vi "外观.vi"(0 "Data In":T1 caption="数据输入", 2 "Display State In":T5={"功能选择"=enum."扫描", "扫描参数"={"+ V"=0.0, "+ Δ V"=0.0, "+ limit I"=0.01, "- V"=0.0, "- Δ V"=0.0, "- limit I"=0.01, "NPLC"=0.001, "模型"=FALSE}, "保持时间"={"V"=0.0, "limit I"=0.01, "T"=0.0, "ΔT"=0.0, "NPLC"=0.001}, "脉冲1"={"t0"=timestamp(0 s since 1904-01-01), "dt"=1.0, "Y"=[]}, "脉冲2"={"t0"=timestamp(0 s since 1904-01-01), "dt"=1.0, "Y"=[]}, "高速脉冲1"={"t0"=timestamp(0 s since 1904-01-01), "dt"=1.0, "Y"=[]}, "高速脉冲2"={"t0"=timestamp(0 s since 1904-01-01), "dt"=1.0, "Y"=[]}, "任意波形"={"t0"=timestamp(0 s since 1904-01-01), "dt"=1.0, "Y"=[]}} caption="显示状态输入" {"保持时间"."ΔT" min=0.5 max=100.0 step=0.1 format="%#_6ps"; "保持时间"."T" min=10.0 max=4294000.0 step=1.0 format="%#_6ps"; "保持时间"."NPLC" min=1.0 max=20.0 step=1.0; "保持时间"."limit I" min=1e-08 max=3.0 format="%#_6pA"; "保持时间"."V" min=-40.0 max=40.0 format="%#_6pV"; "扫描参数"."NPLC" min=0.001 max=25.0 step=0.001; "扫描参数"."- Δ V" min=5e-05 max=1.0 step=5e-05 format="%#_6pV"; "扫描参数"."+ Δ V" min=5e-05 max=1.0 step=5e-05 format="%#_6pV"; "扫描参数"."- V" min=-40.0 max=40.0 format="%#_6pV"; "扫描参数"."- limit I" min=1e-08 max=3.0 format="%#_6pA"; "扫描参数"."+ limit I" min=1e-08 max=3.0 format="%#_6pA"; "扫描参数"."+ V" min=-40.0 max=40.0 format="%#_6pV"}, 3 "Container State":T6 caption="容器状态") -> (6 "Data Out":T1 caption="数据输出", 7 "Display State Out":T5={"功能选择"=enum."扫描", "扫描参数"={"+ V"=0.0, "+ Δ V"=0.0, "+ limit I"=0.01, "- V"=0.0, "- Δ V"=0.0, "- limit I"=0.01, "NPLC"=0.001, "模型"=FALSE}, "保持时间"={"V"=0.0, "limit I"=0.01, "T"=0.0, "ΔT"=0.0, "NPLC"=0.001}, "脉冲1"={"t0"=timestamp(0 s since 1904-01-01), "dt"=1.0, "Y"=[]}, "脉冲2"={"t0"=timestamp(0 s since 1904-01-01), "dt"=1.0, "Y"=[]}, "高速脉冲1"={"t0"=timestamp(0 s since 1904-01-01), "dt"=1.0, "Y"=[]}, "高速脉冲2"={"t0"=timestamp(0 s since 1904-01-01), "dt"=1.0, "Y"=[]}, "任意波形"={"t0"=timestamp(0 s since 1904-01-01), "dt"=1.0, "Y"=[]}} caption="显示状态输出" {"保持时间"."ΔT" min=0.5 max=100.0 step=0.1 format="%#_6ps"; "保持时间"."T" min=10.0 max=4294000.0 step=1.0 format="%#_6ps"; "保持时间"."NPLC" min=1.0 max=20.0 step=1.0; "保持时间"."limit I" min=1e-08 max=3.0 format="%#_6pA"; "保持时间"."V" min=-40.0 max=40.0 format="%#_6pV"; "扫描参数"."NPLC" min=0.001 max=25.0 step=0.001; "扫描参数"."- Δ V" min=5e-05 max=1.0 step=5e-05 format="%#_6pV"; "扫描参数"."+ Δ V" min=5e-05 max=1.0 step=5e-05 format="%#_6pV"; "扫描参数"."- V" min=-40.0 max=40.0 format="%#_6pV"; "扫描参数"."- limit I" min=1e-08 max=3.0 format="%#_6pA"; "扫描参数"."+ limit I" min=1e-08 max=3.0 format="%#_6pA"; "扫描参数"."+ V" min=-40.0 max=40.0 format="%#_6pV"}, 8 "Action":T4 caption="动作")   [LabVIEW 2020, in "功能选择.xctl"]
uses:
  <vilib>/_xctls/Container State.ctl
  <vilib>/_xctls/Action.ctl
  <vilib>/_xctls/XControlSupport.lvlib
panel:
  in  "功能选择":T1
  out "选项卡控件":enum32{"扫描", "保持时间", "脉冲", "高速脉冲", "任意波形"}(tab)
  in  "扫描参数":T2={"+ V"=1.0, "+ Δ V"=0.01, "+ limit I"=0.01, "- V"=1.0, "- Δ V"=0.01, "- limit I"=0.01, "NPLC"=1.0, "模型"=FALSE} {"NPLC" min=0.001 max=25.0 step=0.001; "- Δ V" min=5e-05 max=1.0 step=5e-05 format="%#_6pV"; "+ Δ V" min=5e-05 max=1.0 step=5e-05 format="%#_6pV"; "- V" min=-40.0 max=40.0 format="%#_6pV"; "- limit I" min=1e-08 max=3.0 format="%#_6pA"; "+ limit I" min=1e-08 max=3.0 format="%#_6pA"; "+ V" min=-40.0 max=40.0 format="%#_6pV"}
  in  "保持时间":T3={"V"=0.1, "limit I"=0.01, "T"=10000.0, "ΔT"=1.0, "NPLC"=1.0} {"ΔT" min=0.5 max=100.0 step=0.1 format="%#_6ps"; "T" min=10.0 max=4294000.0 step=1.0 format="%#_6ps"; "NPLC" min=1.0 max=20.0 step=1.0; "limit I" min=1e-08 max=3.0 format="%#_6pA"; "V" min=-40.0 max=40.0 format="%#_6pV"}
  out "脉冲2":waveform(dbl)(graph)
  out "脉冲1":waveform(dbl)(graph)
  out "高速脉冲2":waveform(dbl)(graph) caption="脉冲2"
  out "高速脉冲1":waveform(dbl)(graph) caption="脉冲1"
  out "任意波形":waveform(dbl)(graph)
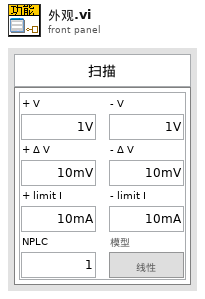
[diagram p1: front panel]
types:
  T1 = typedef "功能选择.xctl/功能类型选择.ctl" = enum16{"扫描", "循环扫描", "保持时间", "脉冲", "高速脉冲", "任意波形"}
  T2 = typedef "功能选择.xctl/扫描参数.ctl" = cluster{"+ V":dbl, "+ Δ V":dbl, "+ limit I":dbl, "- V":dbl, "- Δ V":dbl, "- limit I":dbl, "NPLC":dbl, "模型":bool}
  T3 = typedef "功能选择.xctl/保持时间.ctl" = cluster{"V":dbl, "limit I":dbl, "T":dbl, "ΔT":dbl, "NPLC":dbl}
  T4 = typedef "XControlSupport.lvlib/Action.ctl" = cluster{"Data Changed?":bool, "State Changed?":bool, "Action Name":string}
  T5 = typedef "功能选择.xctl/状态.ctl" = cluster{"功能选择":T1, "扫描参数":T2, "保持时间":T3, "脉冲1":waveform(dbl), "脉冲2":waveform(dbl), "高速脉冲1":waveform(dbl), "高速脉冲2":waveform(dbl), "任意波形":waveform(dbl)}
  T6 = typedef "XControlSupport.lvlib/Container State.ctl" = cluster{"Indicator?":bool, "Run Mode?":bool, " Refnum":refnum<vi>}
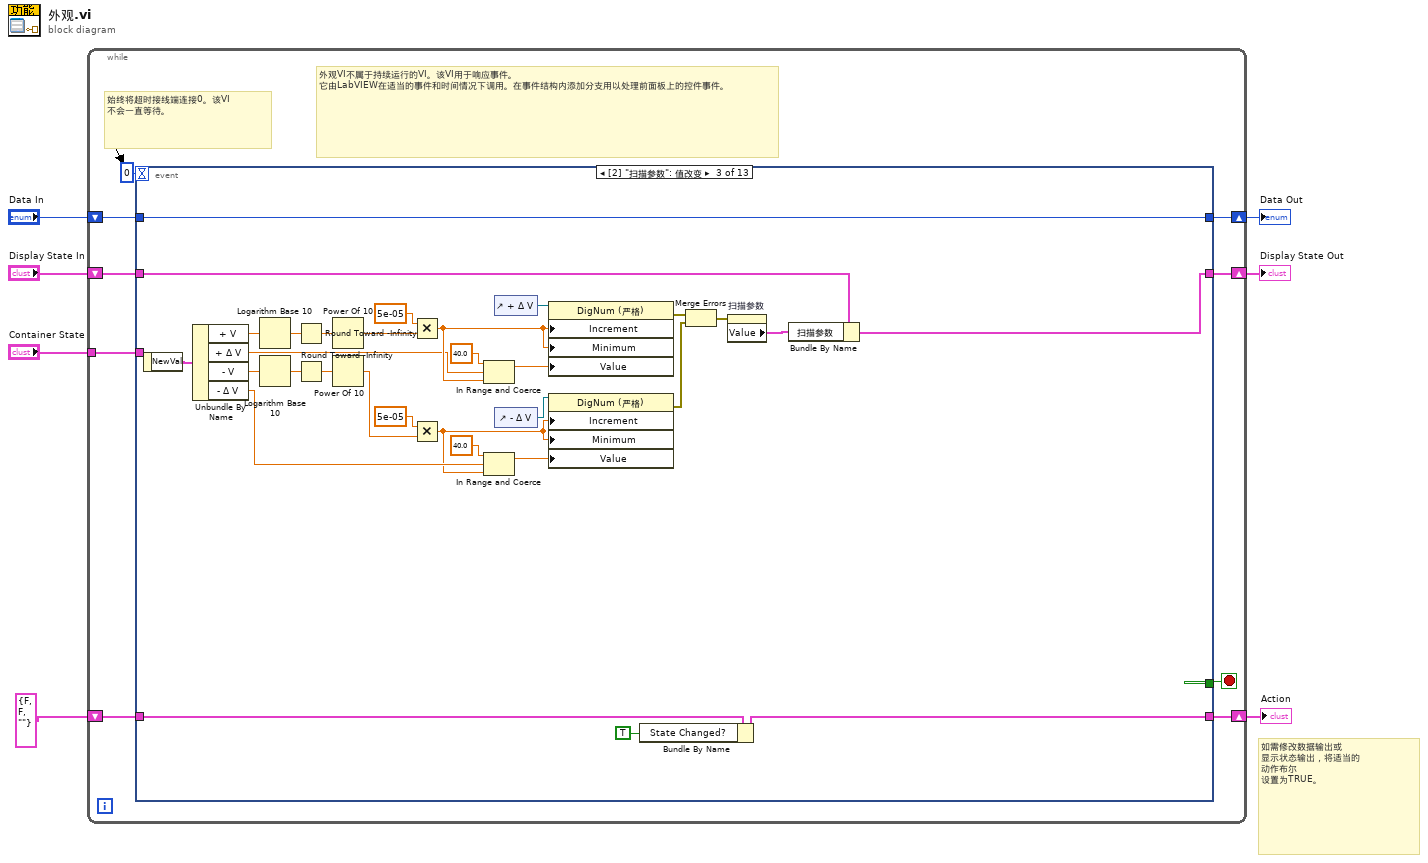
[diagram p0: block diagram]
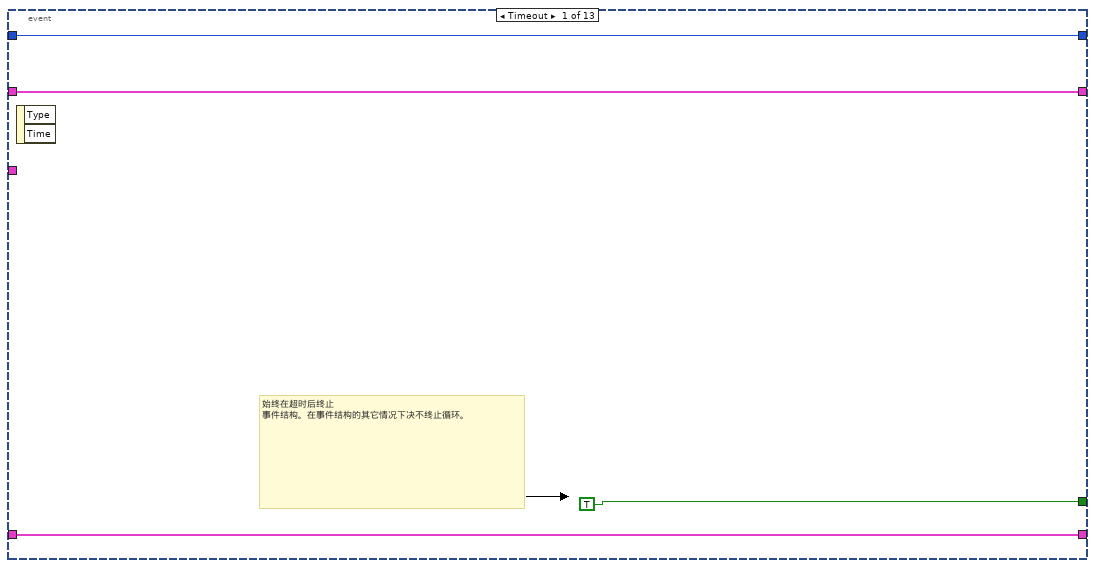
[diagram p2: hidden frame]
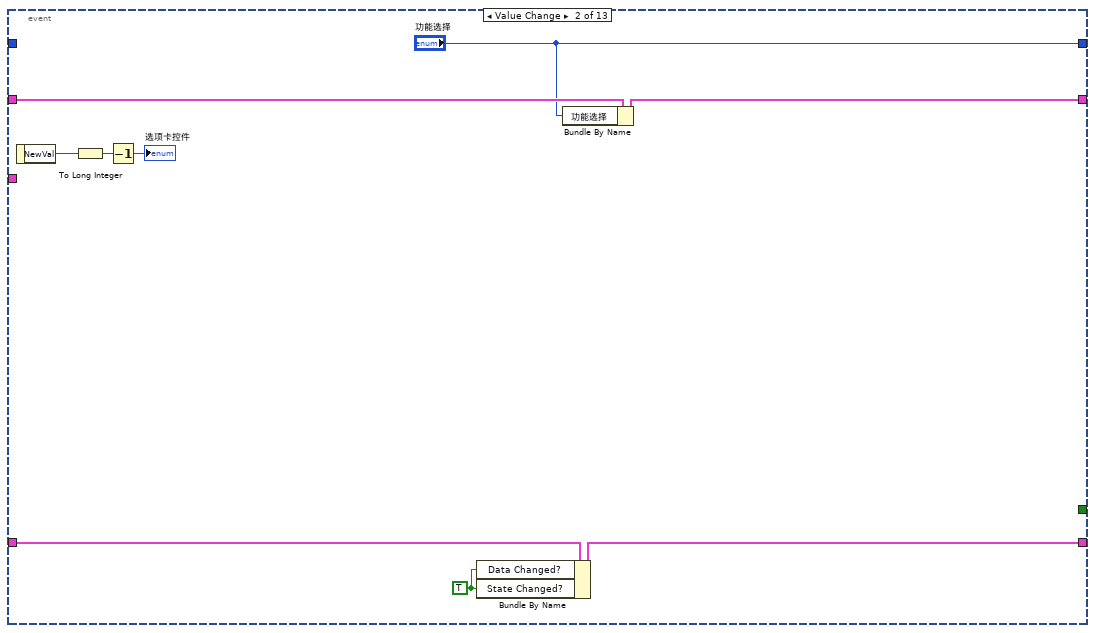
[diagram p3: hidden frame]
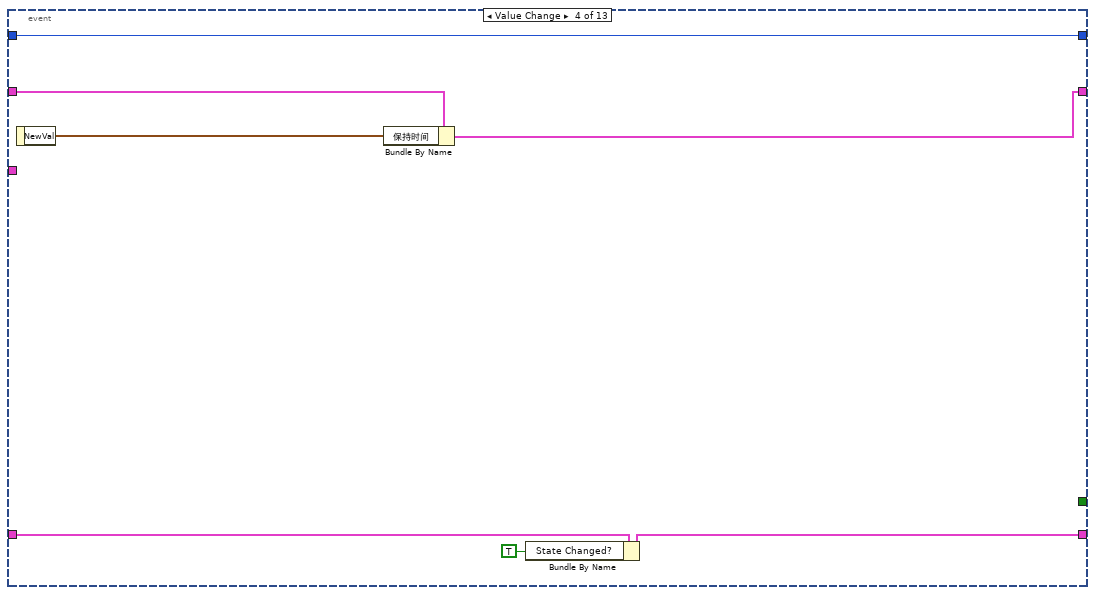
[diagram p4: hidden frame]
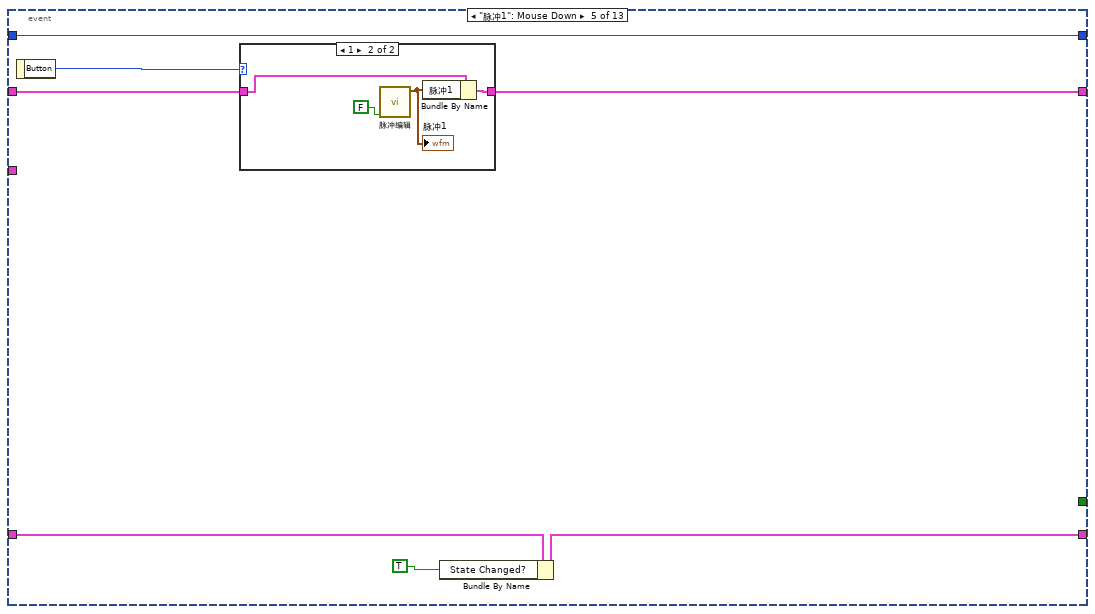
[diagram p5: hidden frame]
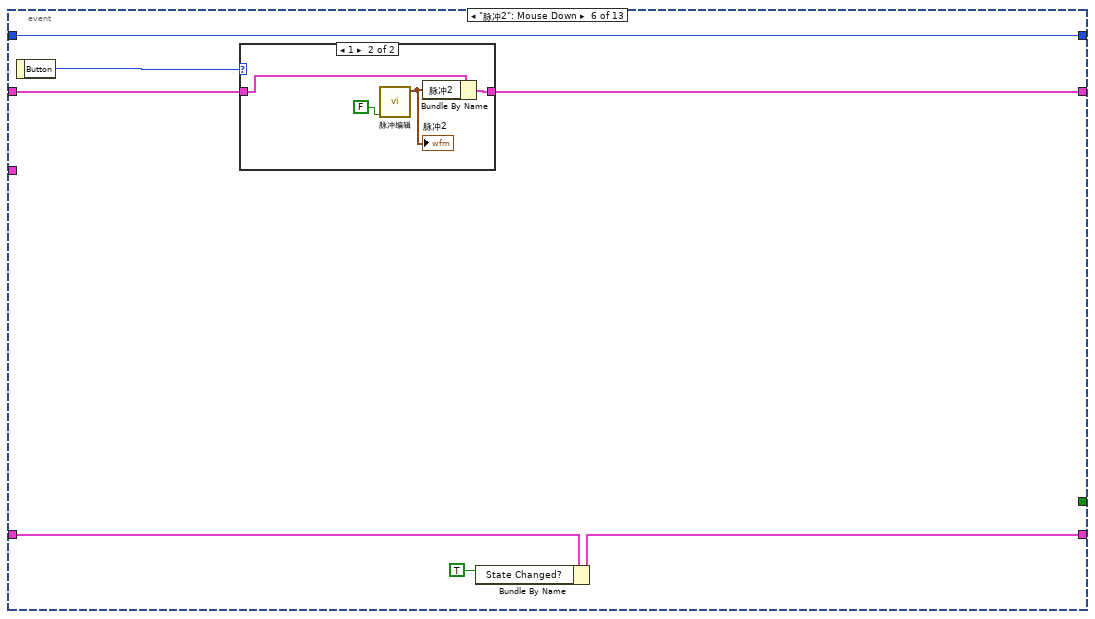
[diagram p7: hidden frame]
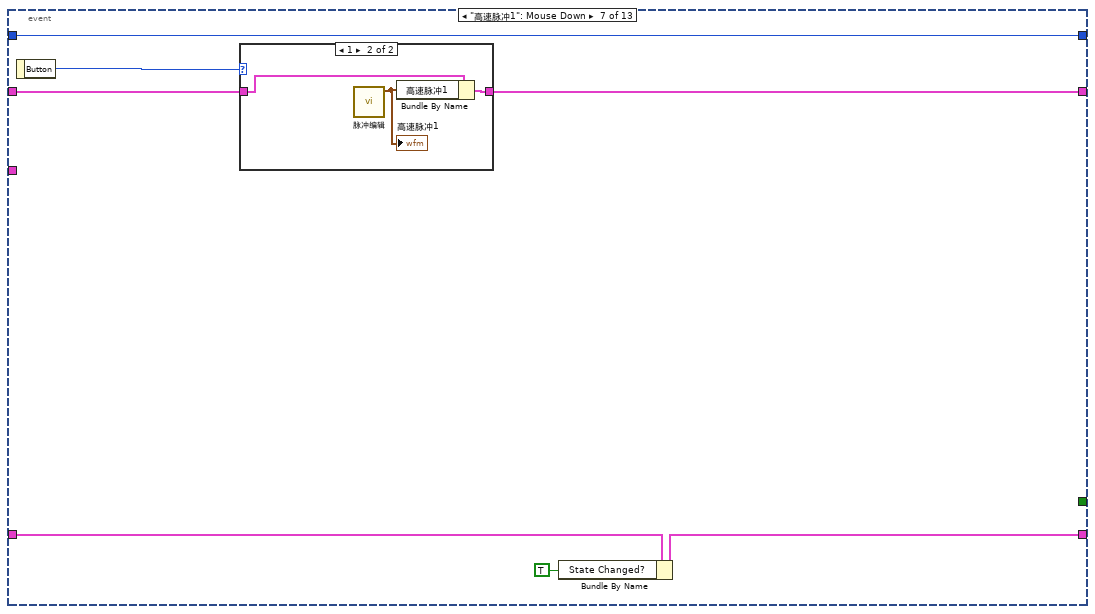
[diagram p9: hidden frame]
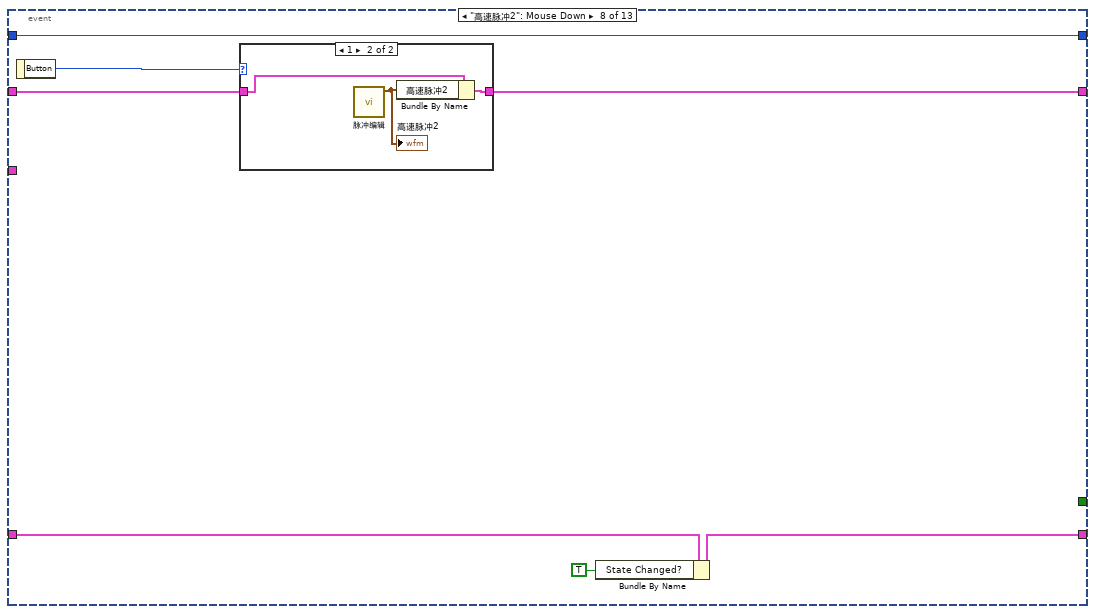
[diagram p11: hidden frame]
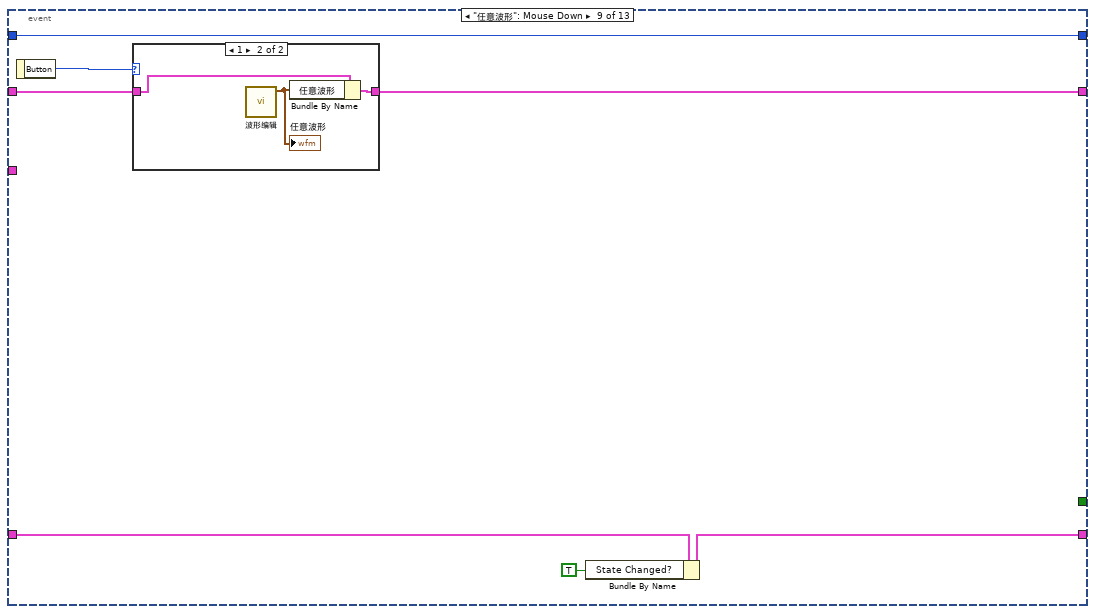
[diagram p13: hidden frame]
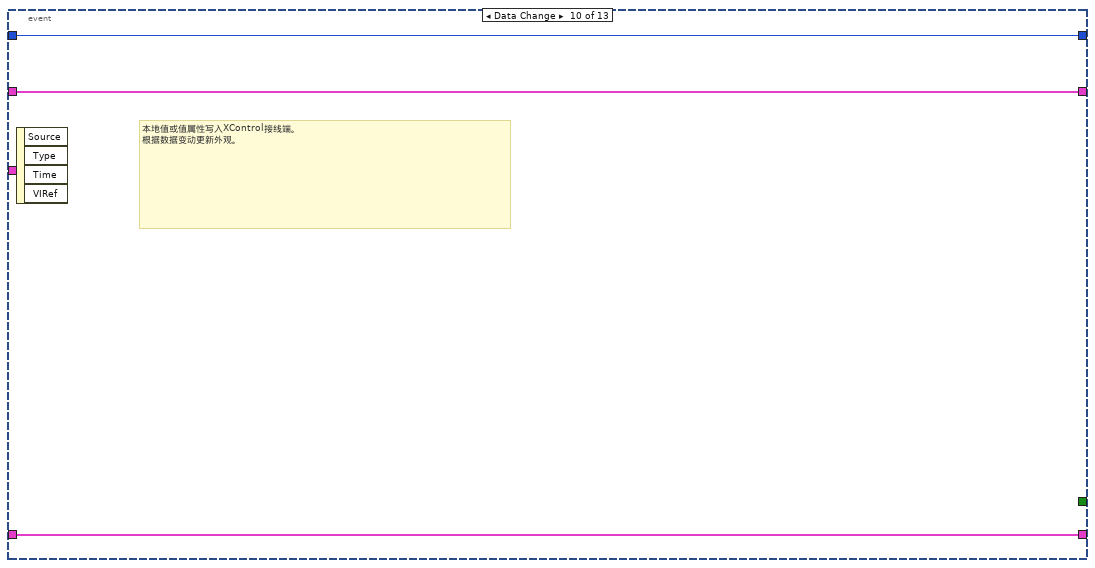
[diagram p15: hidden frame]
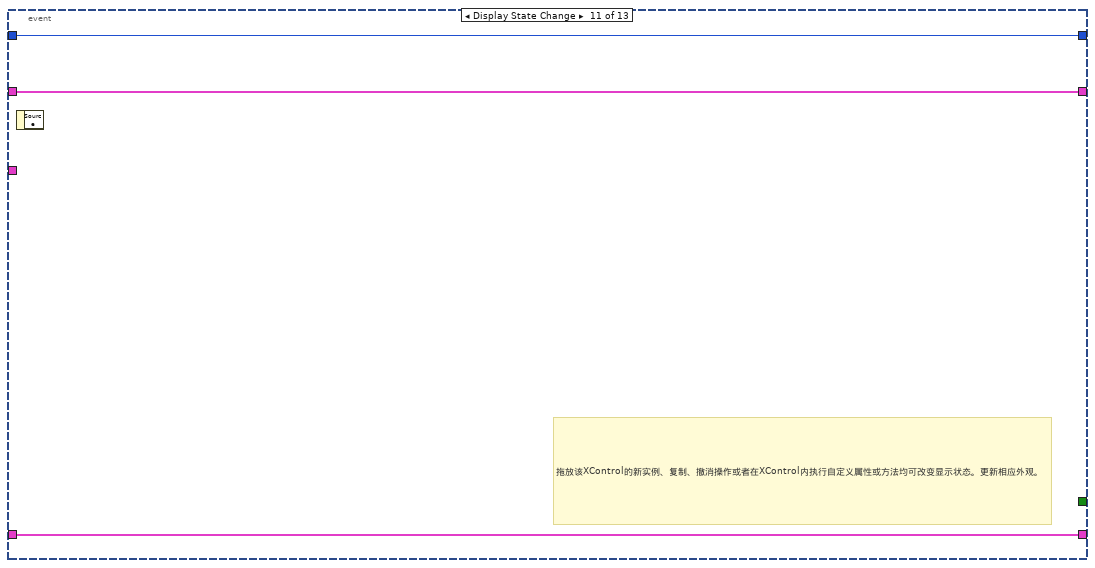
[diagram p16: hidden frame]
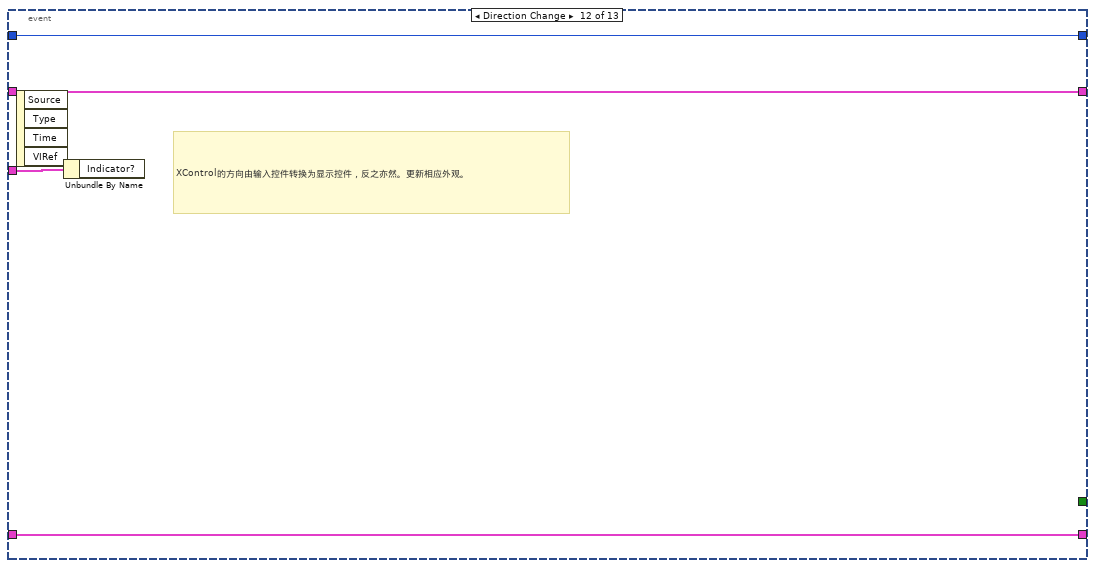
[diagram p17: hidden frame]
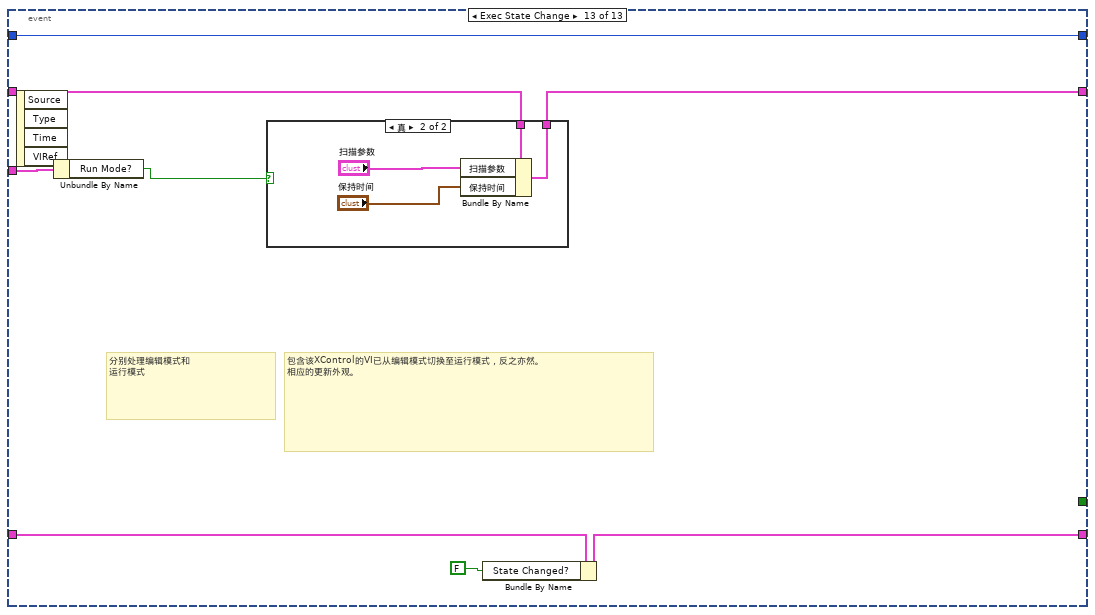
[diagram p18: hidden frame]
diagram:
  # "如需修改数据输出或\n显示状态输出，将适当的\n动作布尔\n设置为TRUE。"
  n1 = while {
    shift-right: [w15] -> w4
    shift-left: "Display State In" -> [w16]
    tunnel: "Container State" -> [w12]
    shift-right: [w10] -> w7
    shift-left: "Data In" -> [w11]
    shift-right: [w8] -> w2
    shift-left: T4 {"Data Changed?"=FALSE, "State Changed?"=FALSE, "Action Name"=""} ("Action") -> [w9]
    stop <- w14 stop-if-true
    # "外观VI不属于持续运行的VI。该VI用于响应事件。  它由LabVIEW在适当的事件和时间情况下调用。在事件结构内添加分支用以处理前面板上的控件事件。"
    # "始终将超时接线端连接0。该VI\n不会一直等待。"
    n2 = event shown="[2] \"扫描参数\": 值改变" {
      selector: _ -> [_ _ _ _ _ _ _ _ _ _ _ _ _]
      dyn-events: _ -> [_ _ _ _ _ _ _ _ _ _ _ _ _]
      timeout: 0 -> [_ _ _ _ _ _ _ _ _ _ _ _ _]
      tunnel: w16 -> [w18 w29 w60 w67 w72 w84 w96 w108 w116 w127 w129 w133 w141]
      tunnel: [w18 w25 w47 w63 w70 w82 w94 w106 w117 w127 w129 w133 w138] -> w15
      tunnel: [TRUE _ _ _ _ _ _ _ _ _ _ _ _] -> w14
      tunnel: w12 -> [_ _ _ _ _ _ _ _ _ _ _ w134 w142]
      tunnel: w11 -> [w17 _ w46 w66 w71 w83 w95 w107 w120 w126 w128 w132 w140]
      tunnel: [w17 "功能选择" w46 w66 w71 w83 w95 w107 w120 w126 w128 w132 w140] -> w10
      tunnel: [w19 w27 w31 w62 w69 w81 w93 w104 w115 w125 w130 w131 w136] -> w8
      tunnel: w9 -> [w19 w28 w59 w65 w74 w86 w98 w109 w119 w125 w130 w131 w139]
      event Timeout {
        # "始终在超时后终止\n事件结构。在事件结构的其它情况下决不终止循环。"
        n3 = event-data() -> ()  [unwired: 1 in, 2 out]
      }
      event Value Change {
        w26 = TRUE ("State Changed?")
        n4 = event-data() -> ("NewVal"=w23:T1)  [unwired: 1 in]
        n5 = To Long Integer(number=w23) -> (32bit integer=w21:i32)
        n6 = Decrement(x=w21) -> (x-1=→"选项卡控件":i32)
        n7 = Bundle By Name(cluster=w28, "Data Changed?"=w26, "State Changed?"=w26) -> (w27:T4)
        n8 = Bundle By Name(cluster=w29, "功能选择"="功能选择") -> (w25:T5)
      }
      event Value Change {
        n9 = event-data() -> ("NewVal"=w54:T2)  [unwired: 1 in]
        n10 = Unbundle By Name(w54) -> ("+ V"=w53:dbl, "+ Δ V"=w44:dbl, "- V"=w48:dbl, "- Δ V"=w40:dbl)
        n11 = Logarithm Base 10(1:w53) -> (0:w58:dbl)
        n12 = Logarithm Base 10(1:w48) -> (0:w49:dbl)
        n13 = Round Toward -Infinity(1:w58) -> (0:w57:dbl)
        n14 = Round Toward -Infinity(1:w49) -> (0:w50:dbl)
        n15 = Power Of 10(x=w57) -> (10^x=w55:dbl)
        n16 = Power Of 10(x=w50) -> (10^x=w52:dbl)
        n17 = Multiply(x=5e-05, y=w55) -> (x*y=w45:dbl)
        n18 = Multiply(x=5e-05, y=w52) -> (x*y=w39:dbl)
        n19 = In Range and Coerce(upper limit=40.0 ("上限"), x=w44, lower limit=w45) -> (coerced(x)=w42:dbl)  [unwired: 1 out]
        n20 = In Range and Coerce(upper limit=40.0 ("上限"), x=w40, lower limit=w39) -> (coerced(x)=w38:dbl)  [unwired: 1 out]
        n21 = control-ref of="+ Δ V"() -> (w33:refnum<vi>)
        n22 = control-ref of="- Δ V"() -> (w32:refnum<vi>)
        n23 = property on="属性节点" class="DigNum (严格)"(reference=w33, "Increment"=w45, "Minimum"=w45, "Value"=w42) -> (error out=w36:errorcluster)  [unwired: 1 in, 1 out]
        n24 = property on="属性节点" class="DigNum (严格)"(reference=w32, "Increment"=w39, "Minimum"=w39, "Value"=w38) -> (error out=w34:errorcluster)  [unwired: 1 in, 1 out]
        n25 = Bundle By Name(cluster=w59, "State Changed?"=TRUE) -> (w31:T4)
        n26 = Merge Errors(w36, w34) -> (w35:errorcluster)
        n27 = property on="扫描参数" class="Clust (严格)"(error in=w35) -> ("Value"=w37:T2)  [unwired: 1 in, 2 out]
        n28 = Bundle By Name(cluster=w60, "扫描参数"=w37) -> (w47:T5)
      }
      event Value Change {
        n29 = event-data() -> ("NewVal"=w64:T3)  [unwired: 1 in]
        n30 = Bundle By Name(cluster=w67, "保持时间"=w64) -> (w63:T5)
        n31 = Bundle By Name(cluster=w65, "State Changed?"=TRUE) -> (w62:T4)
      }
      event "脉冲1": Mouse Down {
        n32 = event-data() -> ("Button"=w73:u16)  [unwired: 1 in]
        n33 = case shown="1" w73 {
          tunnel: w72 -> [w75 w79]
          tunnel: [w75 w78] -> w70
          frame 0, Default {
          }
          frame 1 {
            n34 = call "脉冲编辑.vi"("高速？"=FALSE) -> ("波形图"=w77:waveform(dbl))  [unwired: 10 in]
            "脉冲1" <- w77
            n35 = Bundle By Name(cluster=w79, "脉冲1"=w77) -> (w78:T5)
          }
        }
        n36 = Bundle By Name(cluster=w74, "State Changed?"=TRUE ("Data Changed?")) -> (w69:T4)
      }
      event "脉冲2": Mouse Down {
        n37 = event-data() -> ("Button"=w85:u16)  [unwired: 1 in]
        n38 = case shown="1" w85 {
          tunnel: w84 -> [w87 w91]
          tunnel: [w87 w90] -> w82
          frame 0, Default {
          }
          frame 1 {
            n39 = call "脉冲编辑.vi"("高速？"=FALSE ("高速")) -> ("波形图"=w89:waveform(dbl))  [unwired: 10 in]
            "脉冲2" <- w89
            n40 = Bundle By Name(cluster=w91, "脉冲2"=w89) -> (w90:T5)
          }
        }
        n41 = Bundle By Name(cluster=w86, "State Changed?"=TRUE) -> (w81:T4)
      }
      event "高速脉冲1": Mouse Down {
        n42 = event-data() -> ("Button"=w97:u16)  [unwired: 1 in]
        n43 = case shown="1" w97 {
          tunnel: w96 -> [w99 w102]
          tunnel: [w99 w101] -> w94
          frame 0, Default {
          }
          frame 1 {
            n44 = call "脉冲编辑.vi"() -> ("波形图"=w100:waveform(dbl))  [unwired: 11 in]
            "高速脉冲1" <- w100
            n45 = Bundle By Name(cluster=w102, "高速脉冲1"=w100) -> (w101:T5)
          }
        }
        n46 = Bundle By Name(cluster=w98, "State Changed?"=TRUE) -> (w93:T4)
      }
      event "高速脉冲2": Mouse Down {
        n47 = event-data() -> ("Button"=w105:u16)  [unwired: 1 in]
        n48 = case shown="1" w105 {
          tunnel: w108 -> [w110 w113]
          tunnel: [w110 w112] -> w106
          frame 0, Default {
          }
          frame 1 {
            n49 = call "脉冲编辑.vi"() -> ("波形图"=w111:waveform(dbl))  [unwired: 11 in]
            "高速脉冲2" <- w111
            n50 = Bundle By Name(cluster=w113, "高速脉冲2"=w111) -> (w112:T5)
          }
        }
        n51 = Bundle By Name(cluster=w109, "State Changed?"=TRUE) -> (w104:T4)
      }
      event "任意波形": Mouse Down {
        n52 = event-data() -> ("Button"=w118:u16)  [unwired: 1 in]
        n53 = case shown="1" w118 {
          tunnel: w116 -> [w121 w124]
          tunnel: [w121 w122] -> w117
          frame 0, Default {
          }
          frame 1 {
            n54 = call "波形编辑.vi"() -> ("波形图"=w123:waveform(dbl))  [unwired: 11 in]
            "任意波形" <- w123
            n55 = Bundle By Name(cluster=w124, "任意波形"=w123) -> (w122:T5)
          }
        }
        n56 = Bundle By Name(cluster=w119, "State Changed?"=TRUE) -> (w115:T4)
      }
      event Data Change {
        # "本地值或值属性写入XControl接线端。\n根据数据变动更新外观。"
        n57 = event-data() -> ()  [unwired: 1 in, 4 out]
      }
      event Display State Change {
        # "拖放该XControl的新实例、复制、撤消操作或者在XControl内执行自定义属性或方法均可改变显示状态。更新相应外观。"
        n58 = event-data() -> ()  [unwired: 1 in, 1 out]
      }
      event Direction Change {
        # "XControl的方向由输入控件转换为显示控件，反之亦然。更新相应外观。"
        n59 = event-data() -> ()  [unwired: 1 in, 4 out]
        n60 = Unbundle By Name(w134) -> ()  [unwired: 1 out]
      }
      event Exec State Change {
        # "包含该XControl的VI已从编辑模式切换至运行模式，反之亦然。\n相应的更新外观。"
        # "分别处理编辑模式和\n运行模式"
        n61 = event-data() -> ()  [unwired: 1 in, 4 out]
        n62 = Unbundle By Name(w142) -> ("Run Mode?"=w137:bool)
        n63 = case shown="真" w137 {
          tunnel: w141 -> [w143 w147]
          tunnel: [w143 w146] -> w138
          frame False {
          }
          frame True {
            n64 = Bundle By Name(cluster=w147, "扫描参数"="扫描参数", "保持时间"="保持时间") -> (w146:T5)
          }
        }
        n65 = Bundle By Name(cluster=w139, "State Changed?"=FALSE ("Data Changed?")) -> (w136:T4)
      }
    }
  }
  "Display State Out" <- w4
  "Data Out" <- w7
  "Action" <- w2
